vi "Delete Item By Index.vi"(8 "错误输入":errorcluster, 9 "Index":i32, 11 "Listbox Ref":refnum<vi>) -> (0 "错误输出":errorcluster, 3 "Dup Listbox Ref":refnum<vi>)   [LabVIEW 2012, in "Listbox Tool.lvlib"]
uses:
  Listbox Tool.lvlib
  Custom Type/Read and Write Mode.ctl
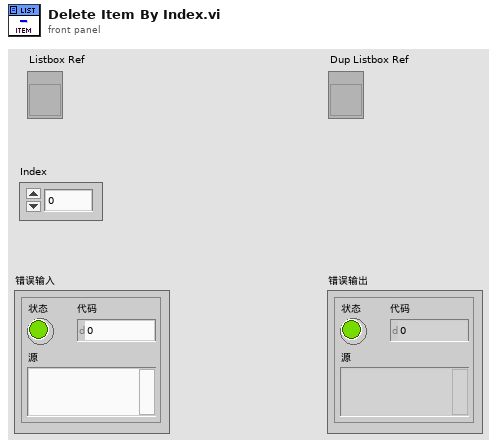
[diagram p1: front panel]
types:
  T1 = typedef "Listbox Tool.lvlib/Read and Write Mode.ctl" = enum16{"Read", "Write"}
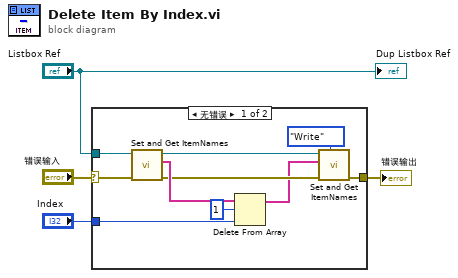
[diagram p0: block diagram]
diagram:
  n1 = case shown="无错误" "错误输入" {
    selector: "错误输入" -> [w14 w15]
    tunnel: "Listbox Ref" -> [w13 _]
    tunnel: "Index" -> [w5 _]
    tunnel: [w8 w15] -> w1
    frame No Error {
      n2 = call "Set and Get ItemNames.vi"("错误输入"=w14, "Listbox Ref"=w13) -> ("错误输出"=w11:errorcluster, "ItemNames Out"=w12:string[], "Dup Listbox Ref"=w10:refnum<vi>)  [unwired: 7 in]
      n3 = Delete From Array(array=w12, length=1 ("长度"), index=w5) -> (array with subset deleted=w7:string[])  [unwired: 1 out]
      n4 = call "Set and Get ItemNames.vi"("Mode"=Read_and_Write_Mode."Write", "错误输入"=w11, "ItemNames In"=w7, "Listbox Ref"=w10) -> ("错误输出"=w8:errorcluster)  [unwired: 5 in, 2 out]
    }
    frame Error {
    }
  }
  "错误输出" <- w1
  "Dup Listbox Ref" <- "Listbox Ref"
